vi "Get Configuration Metadata.vi"(8 "error in (no error)":errorcluster) -> (0 "error out":errorcluster, 3 "Metadata Value":T1(array[cluster]))   [LabVIEW 2020, in "NI-DMM Measurement.lvlib"]
uses:
  NI-DMM Measurement.lvlib
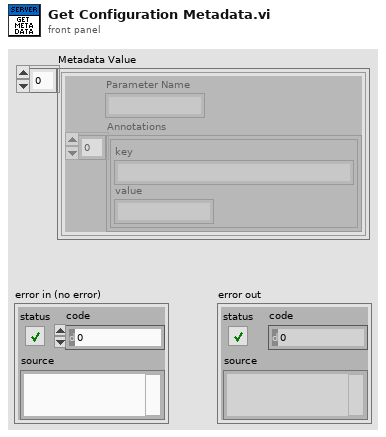
[diagram p1: front panel]
types:
  T1 = cluster{"Parameter Name":string, "Annotations":cluster{"key":string, "value":string}[]}[]
  T2 = typedef "NI-DMM Measurement.lvlib/Parameter Type Specialization.ctl" = cluster{"Parameter Name":string, "Type Specialization":T3, "Annotations":cluster{"Key":T4, "Value":string}[]}
  T3 = typedef "NI-DMM Measurement.lvlib/Type Specialization.ctl" = enum16{"none", "pin"}
  T4 = typedef "NI-DMM Measurement.lvlib/Key.ctl" = enum16{"none", "pin.instrument_type"}
  T5 = cluster{"Parameter Name":string, "Annotations":cluster{"Value":string, "Value 2":string}[]}
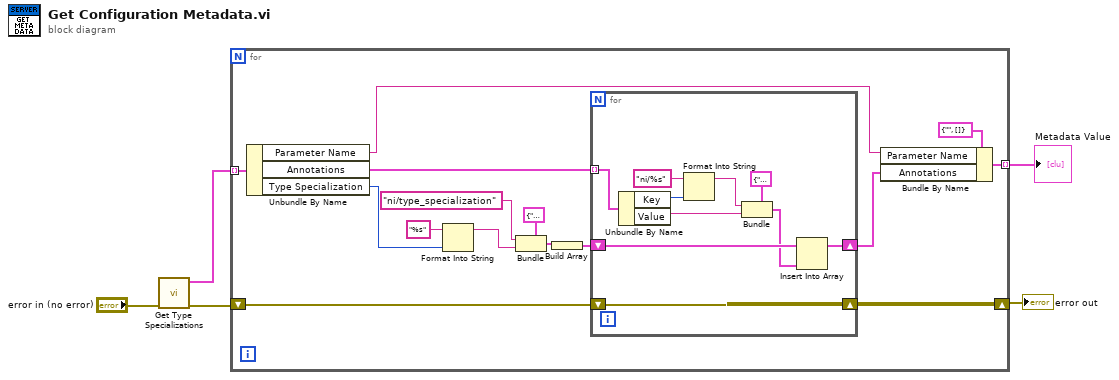
[diagram p0: block diagram]
diagram:
  n1 = call "Get Type Specializations.vi"("error in (no error)"="error in (no error)") -> ("error out"=w1:errorcluster, "Type Specializations"=w2:T2[])  [unwired: 9 in]
  n2 = for {
    tunnel: w2 -> [w20] mode=indexing
    shift-right: [w16] -> w4
    shift-left: w1 -> [w17]
    tunnel: [w18] -> w3 mode=indexing
    n3 = Unbundle By Name(w20) -> ("Parameter Name"=w6:string, "Annotations"=w10:cluster{"Key":T4, "Value":string}[], "Type Specialization"=w14:T3)
    n4 = Format Into String(format string="%s", w14) -> (resulting string=w12:string)  [unwired: 2 in, 1 out]
    n5 = Bundle(cluster=cluster{"Value":string, "Value 2":string} {"Value"="", "Value 2"=""} ("Cluster 2"), "Value"="ni/type_specialization", "Value 2"=w12) -> (w7:cluster{"Value":string, "Value 2":string})
    n6 = Build Array(w7) -> (w8:cluster{"Value":string, "Value 2":string}[])
    n7 = for {
      shift-right: [w30] -> w16
      shift-left: w17 -> [w30]
      tunnel: w10 -> [w29] mode=indexing
      shift-right: [w21] -> w9
      shift-left: w8 -> [w23]
      n8 = Unbundle By Name(w29) -> ("Key"=w27:T4, "Value"=w24:string)
      n9 = Format Into String(format string="ni/%s", w27) -> (resulting string=w25:string)  [unwired: 2 in, 1 out]
      n10 = Bundle(cluster=cluster{"Value":string, "Value 2":string} {"Value"="", "Value 2"=""} ("Cluster 2"), "Value"=w25, "Value 2"=w24) -> (w22:cluster{"Value":string, "Value 2":string})
      n11 = Insert Into Array(array=w23, new element=w22) -> (w21:cluster{"Value":string, "Value 2":string}[])  [unwired: 1 in]
    }
    n12 = Bundle By Name(cluster=T5 {"Parameter Name"="", "Annotations"=[]} ("Cluster"), "Parameter Name"=w6, "Annotations"=w9) -> (w18:T5)
  }
  "error out" <- w4
  "Metadata Value" <- w3
